vi "Change Camera Configuration.vi"(8 "error in (no error)":errorcluster, 10 "Camera Controls":T2={"VideoMode"=81, "Brightness"=150, "Sharpness"=50, "White Balance"=8000, "Saturation"=75, "Exposure"=5} {"VideoMode" items=["640 x 480 YUY 2 30.00 fps", "640 x 480 YUY 2 20.00 fps", "640 x 480 YUY 2 15.00 fps", "640 x 480 YUY 2 10.00 fps", "640 x 480 YUY 2 7.50 fps", "1280 x 720 YUY 2 10.00 fps", "1280 x 720 YUY 2 7.50 fps", "960 x 544 YUY 2 15.00 fps", "960 x 544 YUY 2 10.00 fps", "960 x 544 YUY 2 7.50 fps", "800 x 448 YUY 2 20.00 fps", "800 x 448 YUY 2 15.00 fps", "800 x 448 YUY 2 10.00 fps", "800 x 448 YUY 2 7.50 fps", "640 x 360 YUY 2 30.00 fps", "640 x 360 YUY 2 20.00 fps", "640 x 360 YUY 2 15.00 fps", "640 x 360 YUY 2 10.00 fps", "640 x 360 YUY 2 7.50 fps", "424 x 240 YUY 2 30.00 fps", "424 x 240 YUY 2 20.00 fps", "424 x 240 YUY 2 15.00 fps", "424 x 240 YUY 2 10.00 fps", "424 x 240 YUY 2 7.50 fps", "352 x 288 YUY 2 30.00 fps", "352 x 288 YUY 2 20.00 fps", "352 x 288 YUY 2 15.00 fps", "352 x 288 YUY 2 10.00 fps", "352 x 288 YUY 2 7.50 fps", "320 x 240 YUY 2 30.00 fps", "320 x 240 YUY 2 20.00 fps", "320 x 240 YUY 2 15.00 fps", "320 x 240 YUY 2 10.00 fps", "320 x 240 YUY 2 7.50 fps", "800 x 600 YUY 2 15.00 fps", "800 x 600 YUY 2 10.00 fps", "800 x 600 YUY 2 7.50 fps", "176 x 144 YUY 2 30.00 fps", "176 x 144 YUY 2 20.00 fps", "176 x 144 YUY 2 15.00 fps", "176 x 144 YUY 2 10.00 fps", "176 x 144 YUY 2 7.50 fps", "160 x 120 YUY 2 30.00 fps", "160 x 120 YUY 2 20.00 fps", "160 x 120 YUY 2 15.00 fps", "160 x 120 YUY 2 10.00 fps", "160 x 120 YUY 2 7.50 fps", "1280 x 800 YUY 2 10.00 fps", "640 x 480 JPEG 30.00 fps", "640 x 480 JPEG 20.00 fps", "640 x 480 JPEG 15.00 fps", "640 x 480 JPEG 10.00 fps", "640 x 480 JPEG 7.50 fps", "1280 x 720 JPEG 30.00 fps", "1280 x 720 JPEG 20.00 fps", "1280 x 720 JPEG 15.00 fps", "1280 x 720 JPEG 10.00 fps", "1280 x 720 JPEG 7.50 fps", "960 x 544 JPEG 30.00 fps", "960 x 544 JPEG 20.00 fps", "960 x 544 JPEG 15.00 fps", "960 x 544 JPEG 10.00 fps", "960 x 544 JPEG 7.50 fps", "800 x 448 JPEG 30.00 fps", "800 x 448 JPEG 20.00 fps", "800 x 448 JPEG 15.00 fps", "800 x 448 JPEG 10.00 fps", "800 x 448 JPEG 7.50 fps", "640 x 360 JPEG 30.00 fps", "640 x 360 JPEG 20.00 fps", "640 x 360 JPEG 15.00 fps", "640 x 360 JPEG 10.00 fps", "640 x 360 JPEG 7.50 fps", "800 x 600 JPEG 30.00 fps", "800 x 600 JPEG 20.00 fps", "800 x 600 JPEG 15.00 fps", "800 x 600 JPEG 10.00 fps", "800 x 600 JPEG 7.50 fps", "416 x 240 JPEG 30.00 fps", "416 x 240 JPEG 20.00 fps", "416 x 240 JPEG 15.00 fps", "416 x 240 JPEG 10.00 fps", "416 x 240 JPEG 7.50 fps", "352 x 288 JPEG 30.00 fps", "352 x 288 JPEG 20.00 fps", "352 x 288 JPEG 15.00 fps", "352 x 288 JPEG 10.00 fps", "352 x 288 JPEG 7.50 fps", "176 x 144 JPEG 30.00 fps", "176 x 144 JPEG 20.00 fps", "176 x 144 JPEG 15.00 fps", "176 x 144 JPEG 10.00 fps", "176 x 144 JPEG 7.50 fps", "320 x 240 JPEG 30.00 fps", "320 x 240 JPEG 20.00 fps", "320 x 240 JPEG 15.00 fps", "320 x 240 JPEG 10.00 fps", "320 x 240 JPEG 7.50 fps", "160 x 120 JPEG 30.00 fps", "160 x 120 JPEG 20.00 fps", "160 x 120 JPEG 15.00 fps", "160 x 120 JPEG 10.00 fps", "160 x 120 JPEG 7.50 fps"]}, 11 "Camera Session":T1) -> (0 "error out":errorcluster, 2 "Camera Controls Out":T2={"VideoMode"=81, "Brightness"=150, "Sharpness"=50, "White Balance"=8000, "Saturation"=75, "Exposure"=5} {"VideoMode" items=["640 x 480 YUY 2 30.00 fps", "640 x 480 YUY 2 20.00 fps", "640 x 480 YUY 2 15.00 fps", "640 x 480 YUY 2 10.00 fps", "640 x 480 YUY 2 7.50 fps", "1280 x 720 YUY 2 10.00 fps", "1280 x 720 YUY 2 7.50 fps", "960 x 544 YUY 2 15.00 fps", "960 x 544 YUY 2 10.00 fps", "960 x 544 YUY 2 7.50 fps", "800 x 448 YUY 2 20.00 fps", "800 x 448 YUY 2 15.00 fps", "800 x 448 YUY 2 10.00 fps", "800 x 448 YUY 2 7.50 fps", "640 x 360 YUY 2 30.00 fps", "640 x 360 YUY 2 20.00 fps", "640 x 360 YUY 2 15.00 fps", "640 x 360 YUY 2 10.00 fps", "640 x 360 YUY 2 7.50 fps", "424 x 240 YUY 2 30.00 fps", "424 x 240 YUY 2 20.00 fps", "424 x 240 YUY 2 15.00 fps", "424 x 240 YUY 2 10.00 fps", "424 x 240 YUY 2 7.50 fps", "352 x 288 YUY 2 30.00 fps", "352 x 288 YUY 2 20.00 fps", "352 x 288 YUY 2 15.00 fps", "352 x 288 YUY 2 10.00 fps", "352 x 288 YUY 2 7.50 fps", "320 x 240 YUY 2 30.00 fps", "320 x 240 YUY 2 20.00 fps", "320 x 240 YUY 2 15.00 fps", "320 x 240 YUY 2 10.00 fps", "320 x 240 YUY 2 7.50 fps", "800 x 600 YUY 2 15.00 fps", "800 x 600 YUY 2 10.00 fps", "800 x 600 YUY 2 7.50 fps", "176 x 144 YUY 2 30.00 fps", "176 x 144 YUY 2 20.00 fps", "176 x 144 YUY 2 15.00 fps", "176 x 144 YUY 2 10.00 fps", "176 x 144 YUY 2 7.50 fps", "160 x 120 YUY 2 30.00 fps", "160 x 120 YUY 2 20.00 fps", "160 x 120 YUY 2 15.00 fps", "160 x 120 YUY 2 10.00 fps", "160 x 120 YUY 2 7.50 fps", "1280 x 800 YUY 2 10.00 fps", "640 x 480 JPEG 30.00 fps", "640 x 480 JPEG 20.00 fps", "640 x 480 JPEG 15.00 fps", "640 x 480 JPEG 10.00 fps", "640 x 480 JPEG 7.50 fps", "1280 x 720 JPEG 30.00 fps", "1280 x 720 JPEG 20.00 fps", "1280 x 720 JPEG 15.00 fps", "1280 x 720 JPEG 10.00 fps", "1280 x 720 JPEG 7.50 fps", "960 x 544 JPEG 30.00 fps", "960 x 544 JPEG 20.00 fps", "960 x 544 JPEG 15.00 fps", "960 x 544 JPEG 10.00 fps", "960 x 544 JPEG 7.50 fps", "800 x 448 JPEG 30.00 fps", "800 x 448 JPEG 20.00 fps", "800 x 448 JPEG 15.00 fps", "800 x 448 JPEG 10.00 fps", "800 x 448 JPEG 7.50 fps", "640 x 360 JPEG 30.00 fps", "640 x 360 JPEG 20.00 fps", "640 x 360 JPEG 15.00 fps", "640 x 360 JPEG 10.00 fps", "640 x 360 JPEG 7.50 fps", "800 x 600 JPEG 30.00 fps", "800 x 600 JPEG 20.00 fps", "800 x 600 JPEG 15.00 fps", "800 x 600 JPEG 10.00 fps", "800 x 600 JPEG 7.50 fps", "416 x 240 JPEG 30.00 fps", "416 x 240 JPEG 20.00 fps", "416 x 240 JPEG 15.00 fps", "416 x 240 JPEG 10.00 fps", "416 x 240 JPEG 7.50 fps", "352 x 288 JPEG 30.00 fps", "352 x 288 JPEG 20.00 fps", "352 x 288 JPEG 15.00 fps", "352 x 288 JPEG 10.00 fps", "352 x 288 JPEG 7.50 fps", "176 x 144 JPEG 30.00 fps", "176 x 144 JPEG 20.00 fps", "176 x 144 JPEG 15.00 fps", "176 x 144 JPEG 10.00 fps", "176 x 144 JPEG 7.50 fps", "320 x 240 JPEG 30.00 fps", "320 x 240 JPEG 20.00 fps", "320 x 240 JPEG 15.00 fps", "320 x 240 JPEG 10.00 fps", "320 x 240 JPEG 7.50 fps", "160 x 120 JPEG 30.00 fps", "160 x 120 JPEG 20.00 fps", "160 x 120 JPEG 15.00 fps", "160 x 120 JPEG 10.00 fps", "160 x 120 JPEG 7.50 fps"]}, 3 "Session out":T1)   [LabVIEW 2016]
uses:
  Camera Settings.ctl
  38 Video Mode.ctl
  <vilib>/userdefined/High Color/IMAQdx.ctl
  <resource>/objmgr/imaqdx.rc
  <vilib>/vision/driver/NI_Vision_Acquisition_Software.lvlib
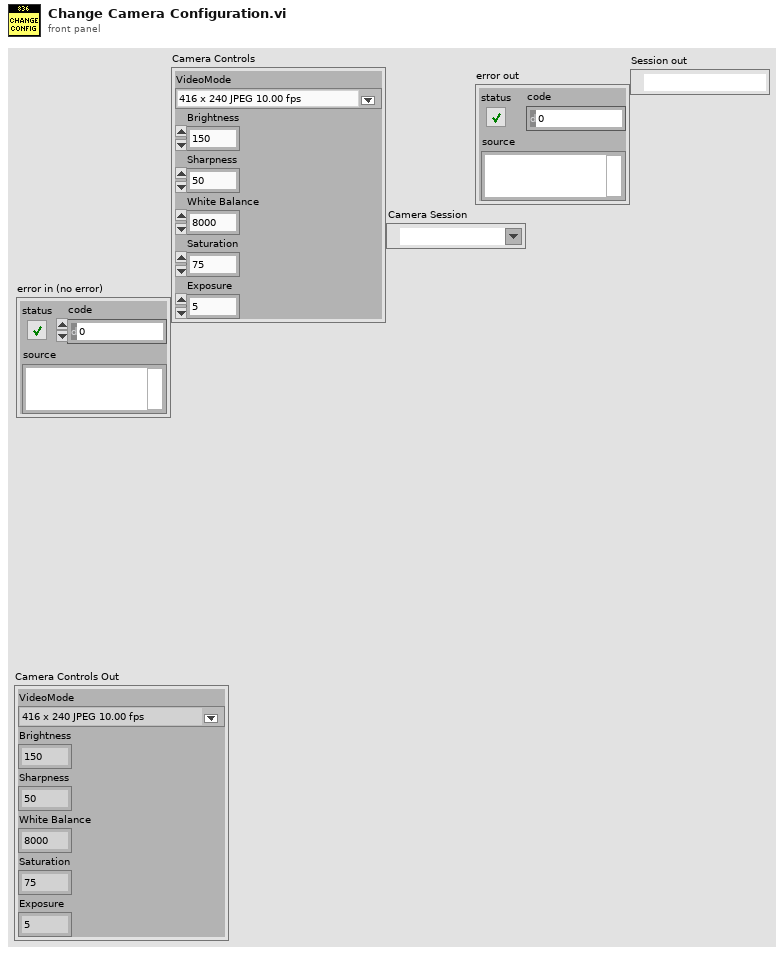
[diagram p1: front panel]
types:
  T1 = typedef "IMAQdx.ctl" = refnum<k21>
  T2 = typedef "Camera Settings.ctl" = cluster{"VideoMode":T3, "Brightness":i64, "Sharpness":i64, "White Balance":i64, "Saturation":i64, "Exposure":i64}
  T3 = typedef "38 Video Mode.ctl" = u32
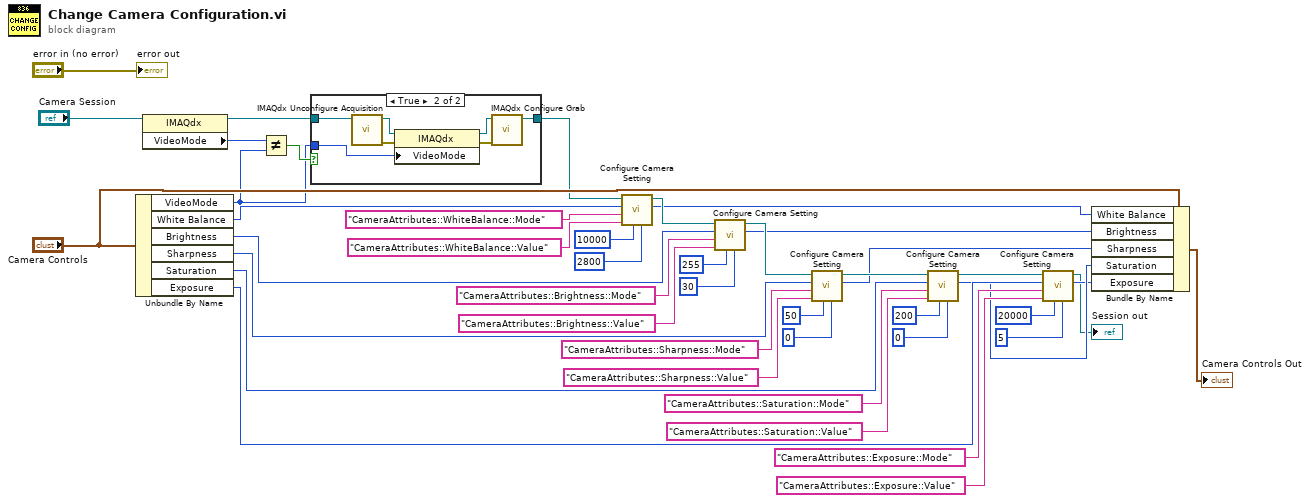
[diagram p0: block diagram]
diagram:
  n1 = Unbundle By Name("Camera Controls") -> ("VideoMode"=w3:T3, "White Balance"=w43:i64, "Brightness"=w42:i64, "Sharpness"=w41:i64, "Saturation"=w40:i64, "Exposure"=w39:i64)
  n2 = property class="IMAQdx"(reference="Camera Session") -> (reference out=w36:T1, "VideoMode"=w34:u32)  [unwired: 1 in, 1 out]
  n3 = Not Equal?(x=w34, y=w3) -> (x != y?=w35:bool)
  n4 = case shown="True" w35 {
    tunnel: w36 -> [w45 w48]
    tunnel: [w45 w47] -> w29
    tunnel: w3 -> [_ w46]
    frame False {
    }
    frame True {
      n5 = call <vilib>:"IMAQdx Unconfigure Acquisition.vi"("Session In"=w48) -> ("error out"=w49:errorcluster, "Session Out"=w52:T1)  [unwired: 9 in]
      n6 = property class="IMAQdx"(reference=w52, error in=w49, "VideoMode"=w46) -> (reference out=w51:T1, error out=w50:errorcluster)
      n7 = call <vilib>:"IMAQdx Configure Grab.vi"("error in"=w50, "Session In"=w51) -> ("Session Out"=w47:T1)  [unwired: 8 in, 1 out]
    }
  }
  n8 = call "Configure Camera Setting.vi"("lower limit"=i64 2800, "upper limit"=i64 10000, 8:"Desired Value"="CameraAttributes::WhiteBalance::Value", "Mode"="CameraAttributes::WhiteBalance::Mode", 10:"Desired Value"=w43, "Session In"=w29) -> ("Set Value"=w9:i64, "Session out"=w26:T1)  [unwired: 4 in]
  n9 = call "Configure Camera Setting.vi"("lower limit"=i64 30, "upper limit"=i64 255, 8:"Desired Value"="CameraAttributes::Brightness::Value", "Mode"="CameraAttributes::Brightness::Mode", 10:"Desired Value"=w42, "Session In"=w26) -> ("Set Value"=w8:i64, "Session out"=w37:T1)  [unwired: 4 in]
  n10 = call "Configure Camera Setting.vi"("lower limit"=i64 0, "upper limit"=i64 50, 8:"Desired Value"="CameraAttributes::Sharpness::Value", "Mode"="CameraAttributes::Sharpness::Mode", 10:"Desired Value"=w41, "Session In"=w37) -> ("Set Value"=w7:i64, "Session out"=w19:T1)  [unwired: 4 in]
  n11 = call "Configure Camera Setting.vi"("lower limit"=i64 0, "upper limit"=i64 200, 8:"Desired Value"="CameraAttributes::Saturation::Value", "Mode"="CameraAttributes::Saturation::Mode", 10:"Desired Value"=w40, "Session In"=w19) -> ("Set Value"=w6:i64, "Session out"=w14:T1)  [unwired: 4 in]
  n12 = call "Configure Camera Setting.vi"("lower limit"=i64 5, "upper limit"=i64 20000, 8:"Desired Value"="CameraAttributes::Exposure::Value", "Mode"="CameraAttributes::Exposure::Mode", 10:"Desired Value"=w39, "Session In"=w14) -> ("Set Value"=w5:i64, "Session out"=→"Session out":T1)  [unwired: 4 in]
  n13 = Bundle By Name(cluster="Camera Controls", "White Balance"=w9, "Brightness"=w8, "Sharpness"=w7, "Saturation"=w6, "Exposure"=w5) -> (→"Camera Controls Out":T2)
  "error out" <- "error in (no error)"
